vi "MyClient_Producer.vi"(8 "error in (no error)":errorcluster, 11 "Stop event":refnum<user-event>) -> (0 "error client source":errorcluster)   [LabVIEW 2018]
uses:
  Client/Client.lvclass/Client.ctl
  Client/Client.lvclass
  C:/Users/jdeboeck/Source/Repos/LV-MQTT-Broker/source/MQTT_Base/MQTT_Base.lvclass
  Control Packets/PUBLISH/PUBLISH.lvclass
  MQTT_Base/MQTT_Base.lvclass
panel:
  out "published":i32
  out "published timer":u32
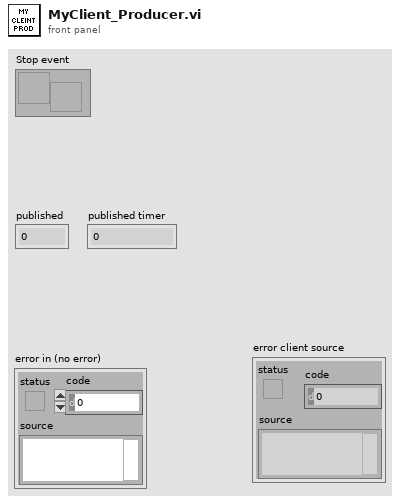
[diagram p1: front panel]
types:
  T1 = typedef "MQTT Server.lvlib/Client.lvclass/Public Events -- cluster.ctl" = cluster{"Connection Status":refnum<user-event>, "Connected":refnum<user-event>, "Application Message":refnum<user-event>}
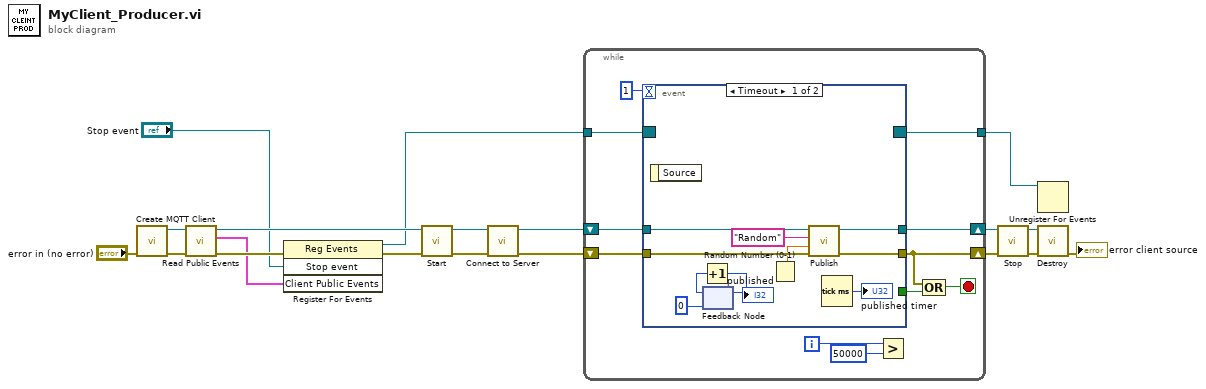
[diagram p0: block diagram]
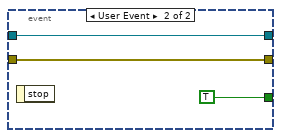
[diagram p2: hidden frame]
diagram:
  n1 = call "Create MQTT Client.vi"("error in (no error)"="error in (no error)") -> ("error out"=w17:errorcluster, "Client out"=w16:refnum<class "Client.lvclass">)  [unwired: 9 in]
  n2 = call "Read Public Events.vi"("error in (no error)"=w17, "Client in"=w16) -> ("error out"=w10:errorcluster, "Client Public Events"=w6:T1, "Client out"=w15:refnum<class "Client.lvclass">)  [unwired: 7 in]
  n3 = register-events(error in=w10, "Stop event", w6) -> (reference out=w8:refnum<event-registration>, error out=w9:errorcluster)  [unwired: 1 in]
  n4 = call "Start.vi"("error in (no error)"=w9, "MQTT_Base in"=w15) -> ("error out"=w3:errorcluster, "MQTT_Base out"=w14:refnum<class "Client.lvclass">)  [unwired: 7 in, 1 out]
  n5 = call "Connect to Server.vi"("error in (no error)"=w3, "Client in"=w14) -> ("error out"=w2:errorcluster, "Client out"=w19:refnum<class "Client.lvclass">)  [unwired: 6 in, 2 out]
  n6 = while {
    shift-right: [w29] -> w13
    shift-left: w19 -> [w30]
    shift-right: [w27] -> w7
    shift-left: w2 -> [w28]
    tunnel: w8 -> [w25]
    tunnel: [w23] -> w5
    i -> [w21]
    stop <- w26 stop-if-true
    n7 = event shown="[0] Timeout" {
      selector: w25 -> [_ _]
      dyn-events: [_ _] -> w23
      timeout: 1 -> [_ _]
      tunnel: w30 -> [w36 w41]
      tunnel: [w35 w41] -> w29
      tunnel: w28 -> [w34 w42]
      tunnel: [w33 w42] -> w27
      tunnel: [_ TRUE] -> w24
      event Timeout {
        n8 = event-data() -> ()  [unwired: 1 in, 1 out]
        n9 = feedback #1(0 ("received")) -> (w39:i32)
        n10 = Increment(x=w39) -> (x+1=w37:i32)
        "published" <- w37
        n11 = feedback-in #1(w37) -> ()
        n12 = Random Number (0-1)() -> (number: 0 to 1=w31:dbl)
        n13 = call "Publish.vi"("error in (no error)"=w34, "Payload"=w31, "Topic Name (empty: Payload name)"="Random", "Client in"=w36) -> ("error out"=w33:errorcluster, "Client out"=w35:refnum<class "Client.lvclass">)  [unwired: 5 in, 1 out]
        n14 = Tick Count (ms)() -> (millisecond timer value=→"published timer":u32)
      }
      event User Event {
        n15 = event-data() -> ()  [unwired: 1 in, 1 out]
      }
    }
    n16 = Greater?(x=w21, y=50000) -> ()  [unwired: 1 out]
    n17 = Compound Arithmetic op=OR(w27, w24) -> (w26:bool)
  }
  n18 = call "Stop.vi"("error in (no error)"=w7, "MQTT_Base in"=w13) -> ("error out"=w11:errorcluster, "MQTT_Base out"=w12:refnum<class "Client.lvclass">)  [unwired: 7 in, 1 out]
  n19 = Unregister For Events(event registration refnum=w5) -> ()  [unwired: 1 in, 1 out]
  n20 = call "Destroy.vi"("error in (no error)"=w11, "MQTT_Base in"=w12) -> ("error out"=→"error client source":errorcluster)  [unwired: 8 in, 1 out]
